vi "FFRead.vi"(1 "pixel":u32=600, 3 "lfkt":i32=1) -> (0 "Data Values":u16[](graph))   [LabVIEW 2014]
uses:
  ESLSCDLL.dll
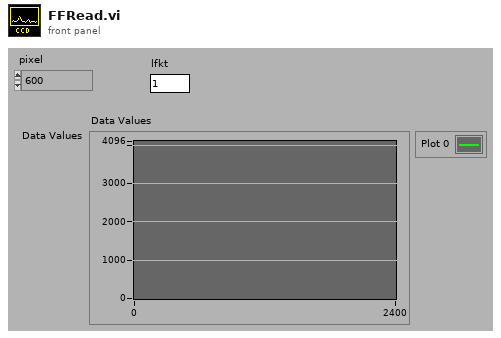
[diagram p1: front panel]
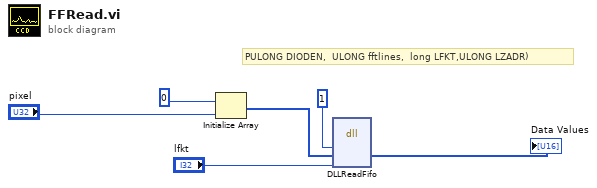
[diagram p0: block diagram]
diagram:
  # "PULONG DIODEN, \tULONG fftlines,  long LFKT,ULONG LZADR)"
  n1 = Initialize Array(u16 0, "pixel") -> (w4:u16[])
  n2 = dll-call lib="C:/Users/Gerhard/Documents/New64/lv/1cam/board.vis/ESLSCDLL.dll" fn="DLLReadFifo"("drv"=u32 1, "dioden"=w4, "fkt"="lfkt") -> ("dioden"=→"Data Values":u16[])  [unwired: 6 in, 2 out]
